vi "To JSON.vi"(11 "ConfigInfoValue in":refnum<class "ConfigInfoValue.lvclass">) -> (2 "JSON string":string)   [LabVIEW 2020, in "Volatus.lvlib" / "ConfigInfoValue.lvclass"]
uses:
  ConfigInfoValue.lvclass
  ConfigInfoValue.lvclass/ConfigInfoValue.ctl
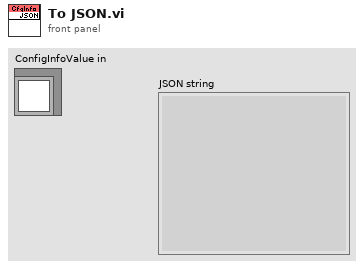
[diagram p1: front panel]
types:
  T1 = cluster{"System":string, "Cluster":string, "Node":string, "Path":string, "Version":string, "Hash":string}
  T2 = typedef "Volatus.lvlib/Config Info.ctl" = cluster{"System":string, "Cluster":string, "Node":string, "Path":path, "Version":string, "Hash":string}
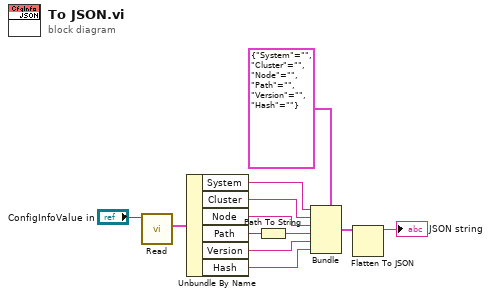
[diagram p0: block diagram]
diagram:
  n1 = call "Read.vi"("ConfigInfoValue in"="ConfigInfoValue in") -> ("Config Info"=w11:T2)  [unwired: 10 in]
  n2 = Unbundle By Name(w11) -> ("System"=w6:string, "Cluster"=w7:string, "Node"=w8:string, "Path"=w10:path, "Version"=w5:string, "Hash"=w4:string)
  n3 = Path To String(path=w10) -> (string=w9:string)
  n4 = Bundle(cluster=T1 {"System"="", "Cluster"="", "Node"="", "Path"="", "Version"="", "Hash"=""}, "System"=w6, "Cluster"=w7, "Node"=w8, "Path"=w9, "Version"=w5, "Hash"=w4) -> (w2:T1)
  n5 = Flatten To JSON(anything=w2) -> (JSON string=→"JSON string":string)  [unwired: 2 in, 1 out]
